vi "YOLO11_Seg_OpenVINO_IR_imgs.vi"() -> ()   [LabVIEW 2018]
doc: "YOLOv8_Seg_OpenVINO_imgs_IR: This example is a semantic segmentation example of the YOLOv8 algorithm, which can call the YOLOv8 object detector and semantic segmentation technology model, and can simultaneously achieve object detection and image semantic segmentation. By combining the target detection performance of the YOLO series with semantic segmentation technology, it is possible to quickly and accurately detect objects in images and segment them into different semantic regions. IR is OpenVINO's proprietary optimized format model."
uses:
  vi.lib/VIRobotics/opencv_yiku/Mat/Mat_8U/Mat_8U.lvclass
  C:/nuc/.package/vi.lib/VIRobotics/opencv_yiku/Mat/Mat/Mat.lvclass
  vi.lib/VIRobotics/ModelZoo/Object_Detection/yolov8_seg_openvino/InitialModel_yolov8_seg_OpenVINO_IR.vi
  vi.lib/VIRobotics/opencv_yiku/Mat/Mat/Mat_release.vi
  vi.lib/VIRobotics/ModelZoo/Object_Detection/yolov8_seg_openvino/yolov8_seg_openvino.lvclass
  vi.lib/VIRobotics/opencv_yiku/opencv_yiku.lvlib
  vi.lib/VIRobotics/opencv_yiku/Mat/Mat/Mat.lvclass
panel:
  in  "device_name":string(combo)="CPU"
  in  "bin_fle":path=path "C:/ProgramData/VIRobotics/ModelZoo/Object_Detection/yolov8_seg/IR_model/yolov8n-seg.bin"
  out "每帧耗时(s)":dbl
  in  "xml_file":path=path "C:/ProgramData/VIRobotics/ModelZoo/Object_Detection/yolov8_seg/IR_model/yolov8n-seg.xml"
  in  "class_names_file":path=path "C:/ProgramData/VIRobotics/ModelZoo/Object_Detection/coco.names"
  out "picture":picture
  in  "imgs":i32(listbox)=1
  in  "image Folder":path=path "C:/ProgramData/VIRobotics/ModelZoo/Object_Detection/imgs"
  in  "stop":bool
  # "Overview: Demonstrates how to read a collection of images and use OpenVINO to  load the IR model of yolo11-seg for real-time image segmentation. \nRequirements: Windows.\nInstructions: \n1.Select the device_name to use.（If your computer has Intel GPU, you can select GPU in the \"type\" control before running the VI to achieve faster inference).\n2.Run the VI.\n3.Click on the image in the imgs control on the right side of the interface that need to be detected.\nIf you want to load the model you trained, follow the following steps:\n1.Select the device_name to use. \n2.Specify the xml_file、bin_file and class_names_file.\n3.Run the VI.\n4.Specify the path of the image Folder and click on the image in the imgs control on the right side of the interface that need to be detected."
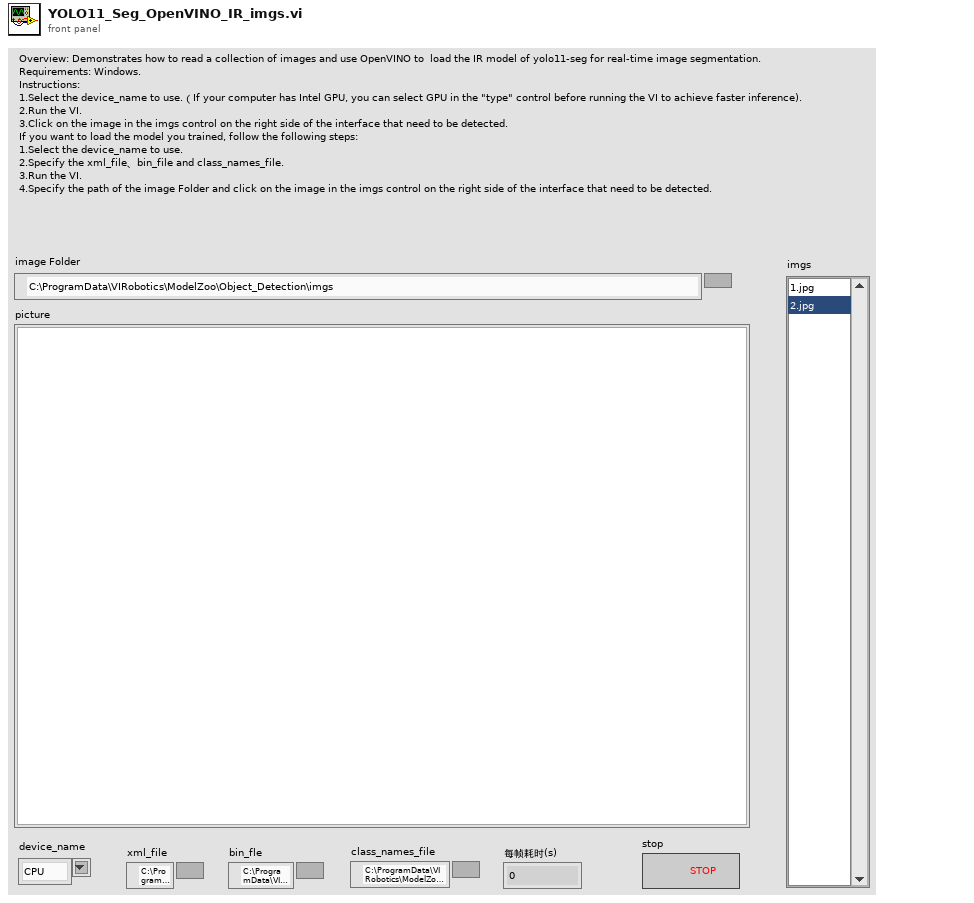
[diagram p1: front panel]
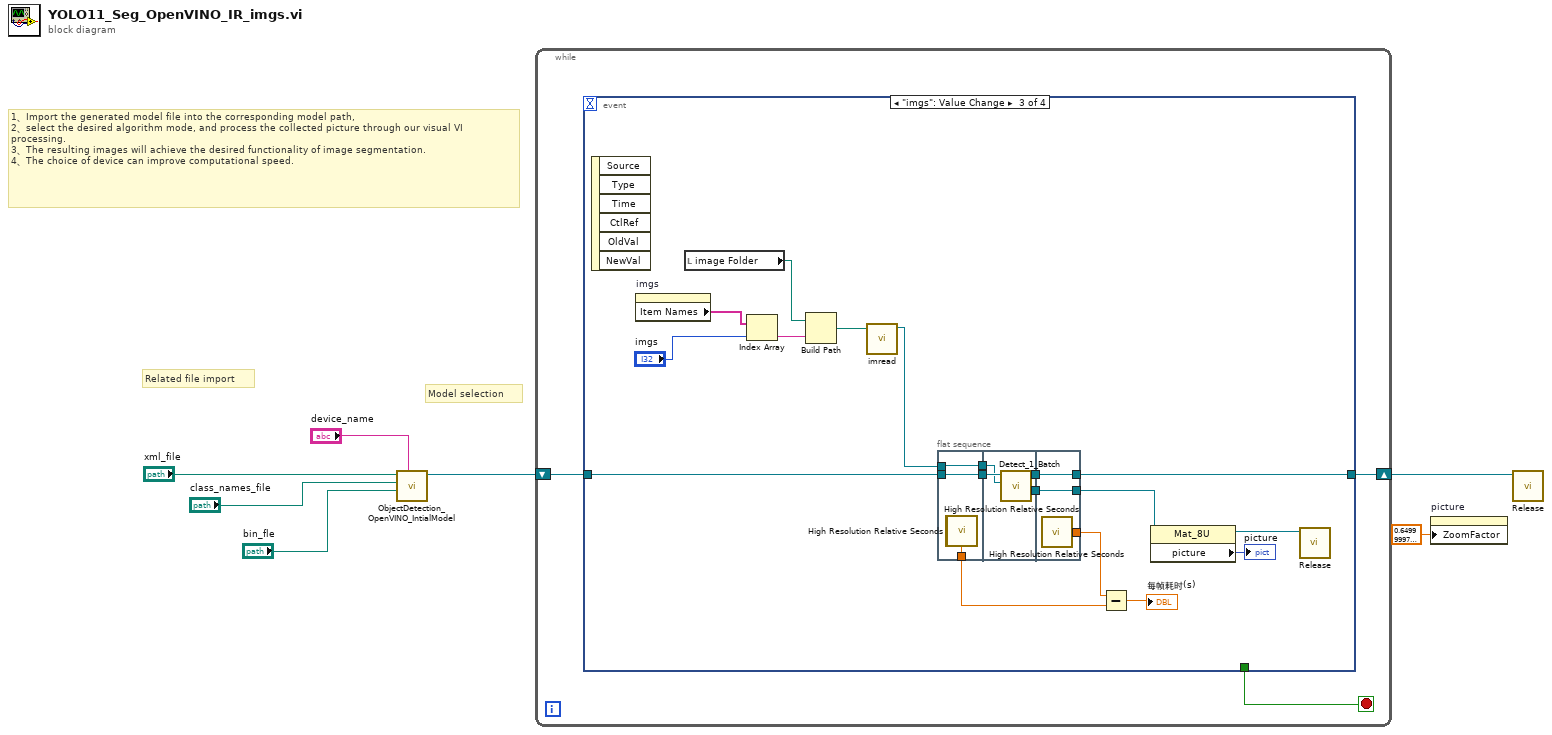
[diagram p0: block diagram]
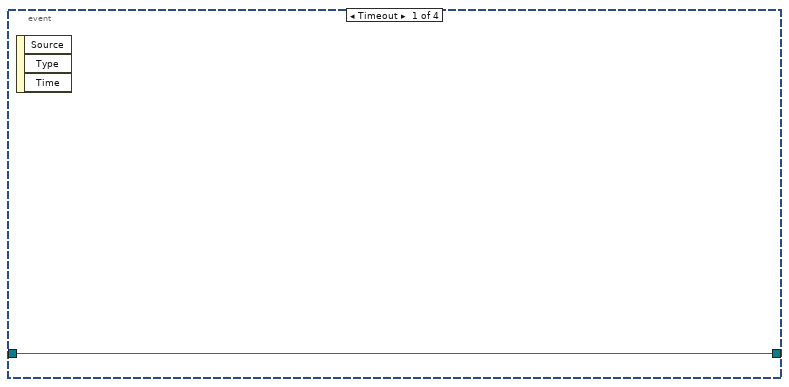
[diagram p2: hidden frame]
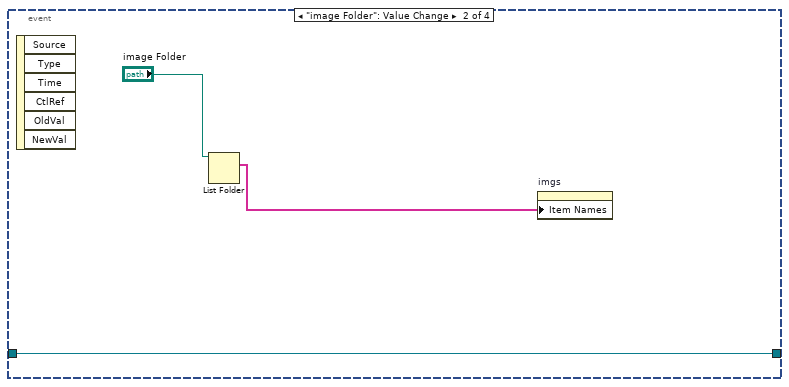
[diagram p3: hidden frame]
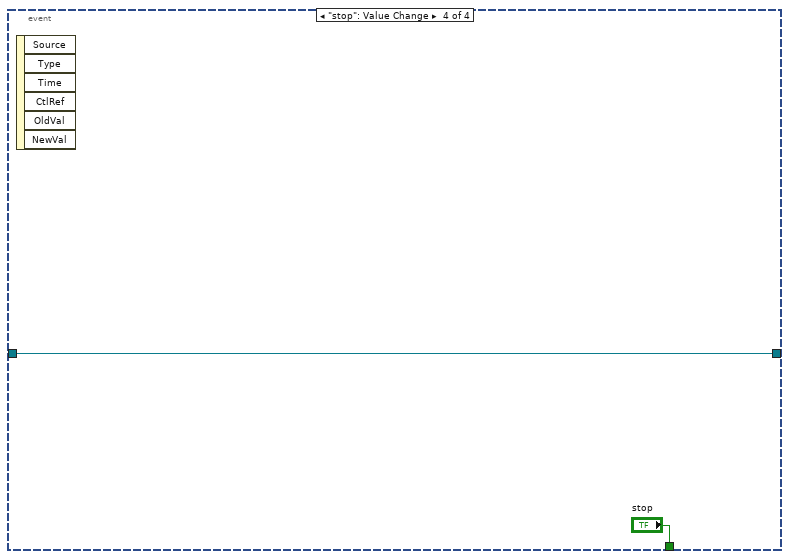
[diagram p4: hidden frame]
diagram:
  # "1、Import the generated model file into the corresponding model path, \n2、select the desired algorithm mode, and process the collected picture through our visual VI processing. \n3、The resulting images will achieve the desired functionality of image segmentation. \n4、The choice of device can improve computational speed."
  # "Related file import"
  # "Model selection"
  n1 = call-poly "ObjectDetection_OpenVINO_IntialModel.vi"("device_name"="device_name", "bin_fle"="bin_fle", "class_names_path"="class_names_file", "xml path"="xml_file") -> ("yolove_seg_openvino out"=w6:refnum<class "yolov8_seg_openvino.lvclass">)  [unwired: 6 in, 1 out]
  n2 = while {
    shift-right: [w9] -> w7
    shift-left: w6 -> [w10]
    stop <- w8 stop-if-true
    n3 = event shown="[2] \"imgs\": Value Change" {
      selector: _ -> [_ _ _ _]
      dyn-events: _ -> [_ _ _ _]
      timeout: _ -> [_ _ _ _]
      tunnel: w10 -> [w11 w12 w27 w43]
      tunnel: [w11 w12 w26 w43] -> w9
      tunnel: [_ _ _ "stop"] -> w8
      event Timeout {
        n4 = event-data() -> ()  [unwired: 1 in, 3 out]
      }
      event "image Folder": Value Change {
        n5 = event-data() -> ()  [unwired: 1 in, 6 out]
        n6 = List Folder(path="image Folder") -> (filenames=w13:string[])  [unwired: 3 in, 3 out]
        n7 = property on="imgs" class="LstBox (strict)"("Item Names"=w13) -> ()  [unwired: 2 in, 2 out]
      }
      event "imgs": Value Change {
        n8 = event-data() -> ()  [unwired: 1 in, 6 out]
        n9 = property on="imgs" class="LstBox (strict)"() -> ("Item Names"=w32:string[])  [unwired: 2 in, 2 out]
        n10 = local read "image Folder"() -> (w29:path)
        n11 = Index Array(array=w32, index="imgs") -> (element=w30:string)
        n12 = Build Path(base path=w29, name or relative path=w30) -> (appended path=w28:path)
        n13 = call "imread.vi"("path"=w28) -> ("Mat out"=w15:refnum<class "Mat_8U.lvclass">)  [unwired: 9 in, 1 out]
        n14 = flat-sequence {
          tunnel: w27 -> [w35]
          tunnel: [w35] -> w22
          tunnel: [w34] -> w18
          tunnel: w15 -> [w33]
          tunnel: [w33] -> w16
          tunnel: w22 -> [w39]
          tunnel: [w38] -> w21
          tunnel: [w37] -> w20
          tunnel: w16 -> [w36]
          tunnel: [w41] -> w25
          tunnel: [w42] -> w26
          tunnel: w21 -> [w42]
          tunnel: w20 -> [w41]
          tunnel: [w40] -> w19
          frame #0 {
            n15 = call <vilib>:"High Resolution Relative Seconds.vi"() -> ("relative seconds"=w34:dbl)
            n16 = call <vilib>:"High Resolution Relative Seconds.vi"() -> ()  [unwired: 1 out]
          }
          frame #1 {
            n17 = call-dynamic "Detect_1_Batch.vi"("image"=w36, "yolov8_seg_openvino in"=w39) -> ("img out"=w37:refnum<class "Mat_8U.lvclass">, "yolov8_seg_openvino out"=w38:refnum<class "yolov8_seg_openvino.lvclass">)  [unwired: 6 in, 2 out]
          }
          frame #2 {
            n18 = call <vilib>:"High Resolution Relative Seconds.vi"() -> ("relative seconds"=w40:dbl)
          }
        }
        n19 = Subtract(x=w19, y=w18) -> (x-y=→"每帧耗时(s)":dbl)
        n20 = property class="Mat_8U"(reference=w25) -> (reference out=w23:refnum<class "Mat_8U.lvclass">, "picture"=→"picture":picture)  [unwired: 1 in, 1 out]
        n21 = call-poly "Release.vi"("Mat in"=w23) -> ()  [unwired: 10 in, 1 out]
      }
      event "stop": Value Change {
        n22 = event-data() -> ()  [unwired: 1 in, 6 out]
      }
    }
  }
  n23 = property on="picture" class="Pict"("ZoomFactor"=sgl 0.65 ("Zoom Factor")) -> ()  [unwired: 2 in, 2 out]
  n24 = call-dynamic "Release.vi"("yolov8_seg_openvino in"=w7) -> ()  [unwired: 9 in, 2 out]
